vi "NIR_Dig.vi"() -> ()   [LabVIEW 2011]
uses:
  <vilib>/DAQmx/write.llb/DAQmx Write (Digital Bool 1Line 1Point).vi
  <vilib>/DAQmx/create/channels.llb/DAQmx Create Channel (DO-Digital Output).vi
  <vilib>/DAQmx/miscellaneous.llb/DAQmx Fill In Error Info.vi
panel:
  in  "NIRLaserOn":bool
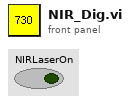
[diagram p1: front panel]
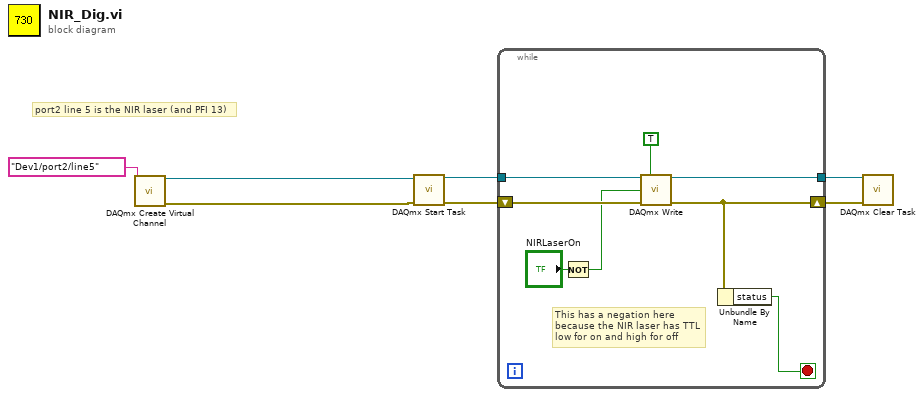
[diagram p0: block diagram]
diagram:
  # "port2 line 5 is the NIR laser (and PFI 13)"
  n1 = call-poly <vilib>:"DAQmx Create Virtual Channel.vi"("lines"=tag "Dev1/port2/line5") -> ("task out"=w2:refnum<k21>, "error out"=w1:errorcluster)  [unwired: 13 in]
  n2 = call <vilib>:"DAQmx Start Task.vi"("task/channels in"=w2, "error in"=w1) -> ("task out"=w7:refnum<k21>, "error out"=w4:errorcluster)  [unwired: 12 in]
  n3 = while {
    tunnel: w7 -> [w15]
    tunnel: [w12] -> w5
    shift-right: [w13] -> w6
    shift-left: w4 -> [w11]
    stop <- w14 stop-if-true
    # "This has a negation here\nbecause the NIR laser has TTL\nlow for on and high for off"
    n4 = Not(x="NIRLaserOn") -> (.not. x?=w8:bool)
    n5 = call-poly <vilib>:"DAQmx Write.vi"("task/channels in"=w15, "auto start"=TRUE, "data"=w8, "error in"=w11) -> ("task out"=w12:refnum<k21>, "error out"=w13:errorcluster)  [unwired: 9 in, 1 out]
    n6 = Unbundle By Name(w13) -> ("status"=w14:bool)
  }
  n7 = call <vilib>:"DAQmx Clear Task.vi"("task in"=w5, "error in"=w6) -> ()  [unwired: 13 in, 1 out]
